vi "experiment.vi"() -> ()   [LabVIEW 2012]
uses:
  <vilib>/DAQmx/create/channels.llb/DAQmx Create Channel (CO-Pulse Generation-Frequency).vi
  <vilib>/DAQmx/configure/timing.llb/DAQmx Timing (Implicit).vi
  <vilib>/Utility/file.llb/Write To Spreadsheet File (DBL).vi
  <vilib>/Analysis/NI_AALBase.lvlib
panel:
  out "Counts":u32=198
  out "After Shelving":T1(graph)
  out "Before Shelving":T1(graph)
  in  "Runs":i32
  in  "shelve for":u32=1000
  in  "dwell after":u32
  in  "deshelve time (ms)":u32
  out "Fraction":dbl
  out "No":i32
  out "Yes":i32
  out "last line":dbl[](array[numeric])
  in  "data file path":path
  in  "stop":bool
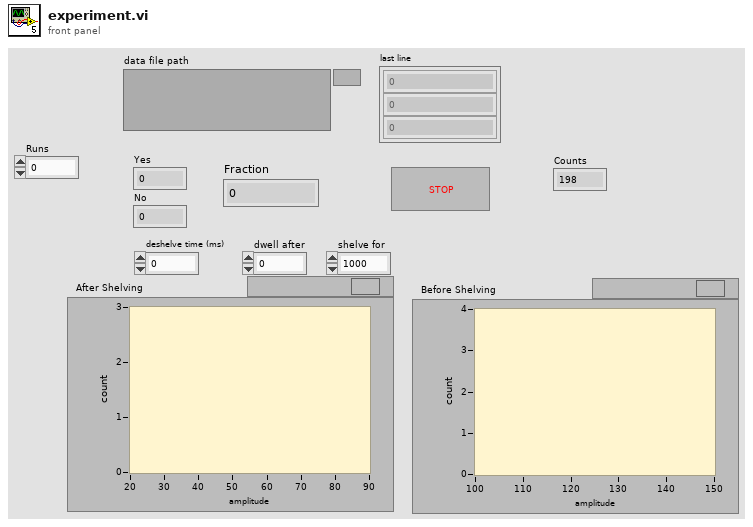
[diagram p1: front panel]
types:
  T1 = cluster{"X Values":dbl[], "Histogram: h(x)":i32[]}
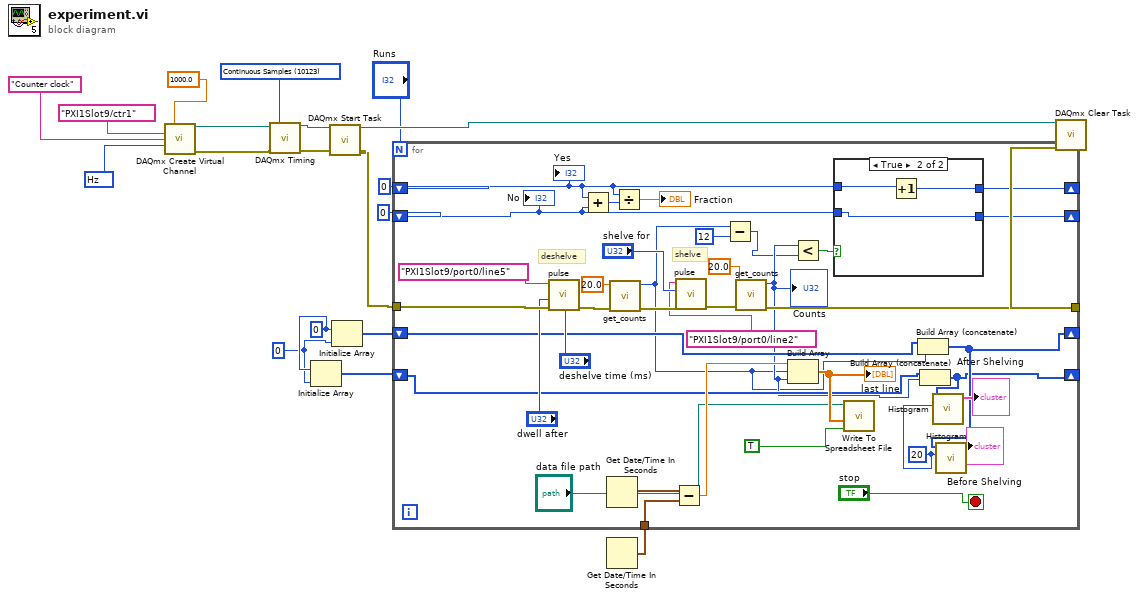
[diagram p0: block diagram]
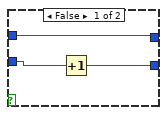
[diagram p2: hidden frame]
diagram:
  w3 = 0 ("dimension size")
  w4 = 0 ("element")
  w15 = 10123 items=["Finite Samples"=10178, "Continuous Samples"=10123, "Hardware Timed Single Point"=12522] ("sample mode")
  w20 = 10373 items=["Hz"=10373] ("units")
  n1 = call-poly <vilib>:"DAQmx Create Virtual Channel.vi"("frequency"=1000.0 ("rate"), "counter"=tag "PXI1Slot9/ctr1", "name to assign"="Counter clock", "units"=w20) -> ("task out"=w19:refnum<k21>, "error out"=w18:errorcluster)  [unwired: 10 in]
  n2 = call-poly <vilib>:"DAQmx Timing.vi"("task/channels in"=w19, "sample mode"=w15, "error in"=w18) -> ("task out"=w17:refnum<k21>, "error out"=w16:errorcluster)  [unwired: 11 in]
  n3 = Initialize Array(w4, w3) -> (w1:i32[])
  n4 = call <vilib>:"DAQmx Start Task.vi"("task/channels in"=w17, "error in"=w16) -> ("task out"=w10:refnum<k21>, "error out"=w11:errorcluster)  [unwired: 12 in]
  n5 = Initialize Array(w4, w3) -> (w2:i32[])
  n6 = Get Date/Time In Seconds() -> (seconds since 1Jan1904=w9:timestamp)
  n7 = for {
    N: "Runs" -> [_]
    tunnel: w11 -> [w56]
    tunnel: w9 -> [w50]
    shift-right: [w45] -> _
    shift-left: 0 -> [w35]
    shift-right: [w44] -> _
    shift-left: 0 -> [w34]
    tunnel: [w37] -> w6
    shift-right: [w25] -> _
    shift-left: w1 -> [w31]
    shift-right: [w26] -> _
    shift-left: w2 -> [w32]
    stop <- "stop" stop-if-true
    w29 = 20 ("intervals")
    # "shelve"
    # "deshelve"
    n8 = call "pulse.vi"("error in"=w56, "dwell after"="dwell after", "time on"="deshelve time (ms)", "lines 2"=tag "PXI1Slot9/port0/line5") -> ("error out"=w57:errorcluster)  [unwired: 3 in]
    n9 = Add(x=w35, y=w34) -> (x+y=w36:i32)
    n10 = Get Date/Time In Seconds() -> (seconds since 1Jan1904=w51:timestamp)
    n11 = call "get_counts.vi"("error in"=w57, "Detection length (ms)"=20.0) -> ("error out"=w55:errorcluster, "Counts"=w23:u32)  [unwired: 8 in]
    n12 = Divide(x=w35, y=w36) -> (x/y=→"Fraction":dbl)
    n13 = Subtract(x=w51, y=w50) -> (x-y=w49:dbl)
    n14 = call "pulse.vi"("error in"=w55, "time on"="shelve for", "lines 2"=tag "PXI1Slot9/port0/line2") -> ("error out"=w54:errorcluster)  [unwired: 4 in]
    n15 = Subtract(x=w23, y=u32 12) -> (x-y=w21:u32)
    n16 = call "get_counts.vi"("error in"=w54, "Detection length (ms)"=20.0) -> ("error out"=w37:errorcluster, "Counts"=w30:u32)  [unwired: 8 in]
    "Counts" <- w30
    n17 = Build Array(w49, w23, w30) -> (w48:dbl[])
    "last line" <- w48
    n18 = Less?(x=w30, y=w21) -> (x < y?=w46:bool)
    n19 = case shown="True" w46 {
      tunnel: w35 -> [w58 w63]
      tunnel: [w58 w62] -> w45
      tunnel: w34 -> [w60 w61]
      tunnel: [w59 w61] -> w44
      frame False {
        n20 = Increment(x=w60) -> (x+1=w59:i32)
      }
      frame True {
        n21 = Increment(x=w63) -> (x+1=w62:i32)
      }
    }
    n22 = call-poly <vilib>:"Write To Spreadsheet File.vi"("append to file? (new file:F)"=TRUE, "1D data"=w48, "file path (dialog if empty)"="data file path") -> ()  [unwired: 5 in, 1 out]
    n23 = Build Array (concatenate)(w32, w23) -> (w26:u32[])
    n24 = Build Array (concatenate)(w31, w30) -> (w25:u32[])
    n25 = call <vilib>:"Histogram.vi"("intervals"=w29, "X"=w25) -> ("Histogram Graph"=→"After Shelving":T1)  [unwired: 6 in, 3 out]
    n26 = call <vilib>:"Histogram.vi"("intervals"=w29, "X"=w26) -> ("Histogram Graph"=→"Before Shelving":T1)  [unwired: 6 in, 3 out]
    "Yes" <- w35
    "No" <- w34
  }
  n27 = call <vilib>:"DAQmx Clear Task.vi"("task in"=w10, "error in"=w6) -> ()  [unwired: 13 in, 1 out]
